vi "Set Configuration.vi"(6 "enabled":bool, 8 "error in (no error)":errorcluster, 9 "unit":T1, 10 "temperature setpoint":dbl, 11 "Temperature Controller in":refnum<class "Temperature Controller.lvclass">) -> (0 "error out":errorcluster, 3 "Temperature Controller out":refnum<class "Temperature Controller.lvclass">)   [LabVIEW 2019, in "Temperature Controller.lvclass"]
uses:
  Temperature Controller.lvclass
  Units.ctl
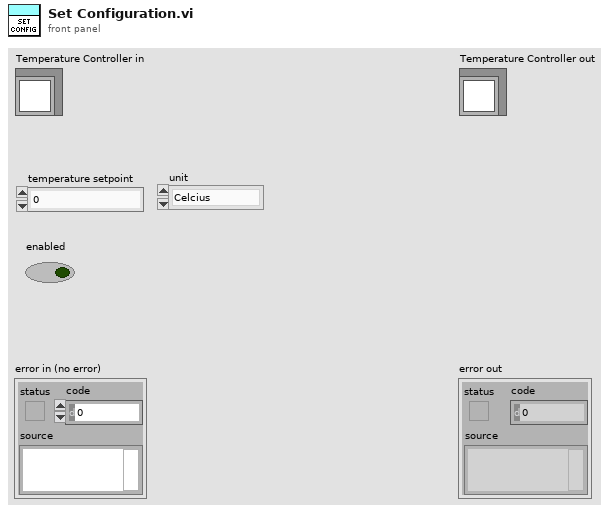
[diagram p1: front panel]
types:
  T1 = typedef "Temperature Controller.lvclass/Units.ctl" = enum16{"Celcius", "Fahrenheit"}
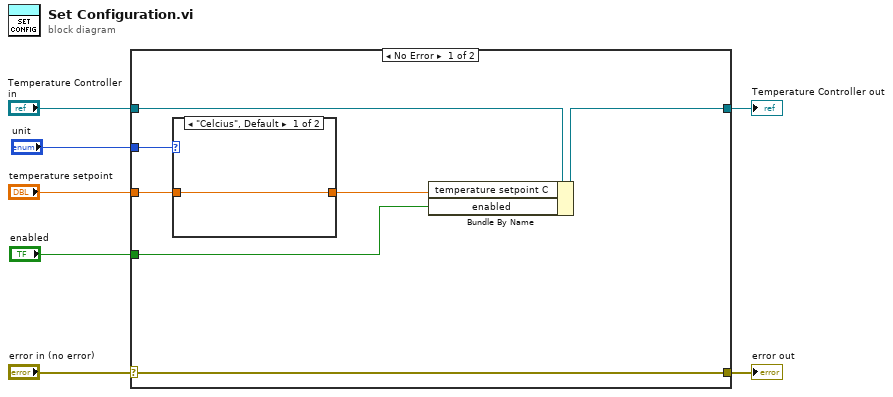
[diagram p0: block diagram]
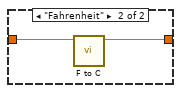
[diagram p2: hidden frame]
diagram:
  n1 = case shown="No Error" "error in (no error)" {
    selector: "error in (no error)" -> [w13 w19]
    tunnel: [w13 w19] -> w6
    tunnel: [w10 w18] -> w4
    tunnel: "Temperature Controller in" -> [w14 w18]
    tunnel: "unit" -> [w12 _]
    tunnel: "temperature setpoint" -> [w11 _]
    tunnel: "enabled" -> [w8 _]
    frame No Error {
      n2 = case shown="\"Celcius\", Default" w12 {
        tunnel: w11 -> [w15 w17]
        tunnel: [w15 w16] -> w9
        frame "Celcius", Default {
        }
        frame "Fahrenheit" {
          n3 = call "F to C.vi"("fahrenheit"=w17) -> ("celsius"=w16:dbl)  [unwired: 10 in]
        }
      }
      n4 = Bundle By Name(cluster=w14, "temperature setpoint C"=w9, "enabled"=w8) -> (w10:refnum<class "Temperature Controller.lvclass">)
    }
    frame Error {
    }
  }
  "error out" <- w6
  "Temperature Controller out" <- w4
